vi "Find adresse RS306.vi"() -> (3 "VISA Resource Name":refnum<visa-resource-name>="TCPIP0::172.20.5.7::inst0::INSTR")   [LabVIEW 2020, in "Library Instrument & Equipement.lvlib" / "Library Spectrum Analyser.lvlib" / "Class Spectrum_Analyser RS306B.lvclass"]
uses:
  Class Spectrum_Analyser RS306B.lvclass
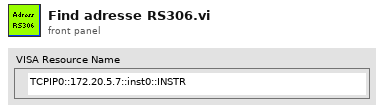
[diagram p1: front panel]
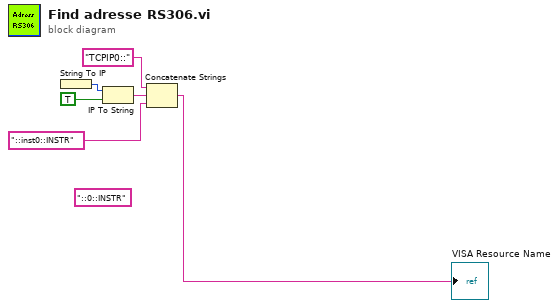
[diagram p0: block diagram]
diagram:
  (unwired) "::0::INSTR"
  n1 = String To IP() -> (0:w6:u32)  [unwired: 1 in]
  n2 = IP To String(1:TRUE ("notation à points ? (F)"), 2:w6) -> (0:w4:string)
  n3 = Concatenate Strings("TCPIP0::", w4, "::inst0::INSTR") -> (→"VISA Resource Name":string)
